vi "CCE MGLD PMJD PF SubVI02.vi"(11 "captura":T2) -> (0 "orientacion correcta":bool, 1 "y":sgl, 2 "x":sgl, 3 "etiqueta detectada":bool, 5 "Image 4":T2(plugin-control))   [LabVIEW 2020]
doc: "Ceballos Conde Emanuel Meneses Gutiérrez Luis David Pineda Méndez Job Daniel 4MV6 Sistemas de visión artificial 2022/1 \nEste vi detecta si se encuentra o no el patrón de la etiqueta ( en este caso la letra pi) en la imagen y devuelve las coordenadas en pixeles del centro de dicho patrón y determina si el patrón se encuentra en la orientación correcta gracias a su ángulo obtenido"
uses:
  <vilib>/vision/Image Controls.llb/IMAQ Image.ctl
  <vilib>/vision/NI_Vision_Development_Module.lvlib
panel:
  out "Angle":sgl
  out "Number of Matches":i32
  out "Matches (real-world)":T1(array[cluster]) {"Bounding Box"."y" format="%.2f"; "Bounding Box"."x" format="%.2f"; "Score" format="%.2f"; "Scale" format="%.2f"; "Angle" format="%.2f"; "Position"."y" format="%.2f"; "Position"."x" format="%.2f"}
  out "patron":T2(plugin-control)
  out "Image 2":T2(plugin-control)
  # "Ceballos Conde Emanuel  Meneses Gutiérrez Luis David  Pineda Méndez Job Daniel 4MV6 Sistemas de visión artificial  2022/1             SubVI02"
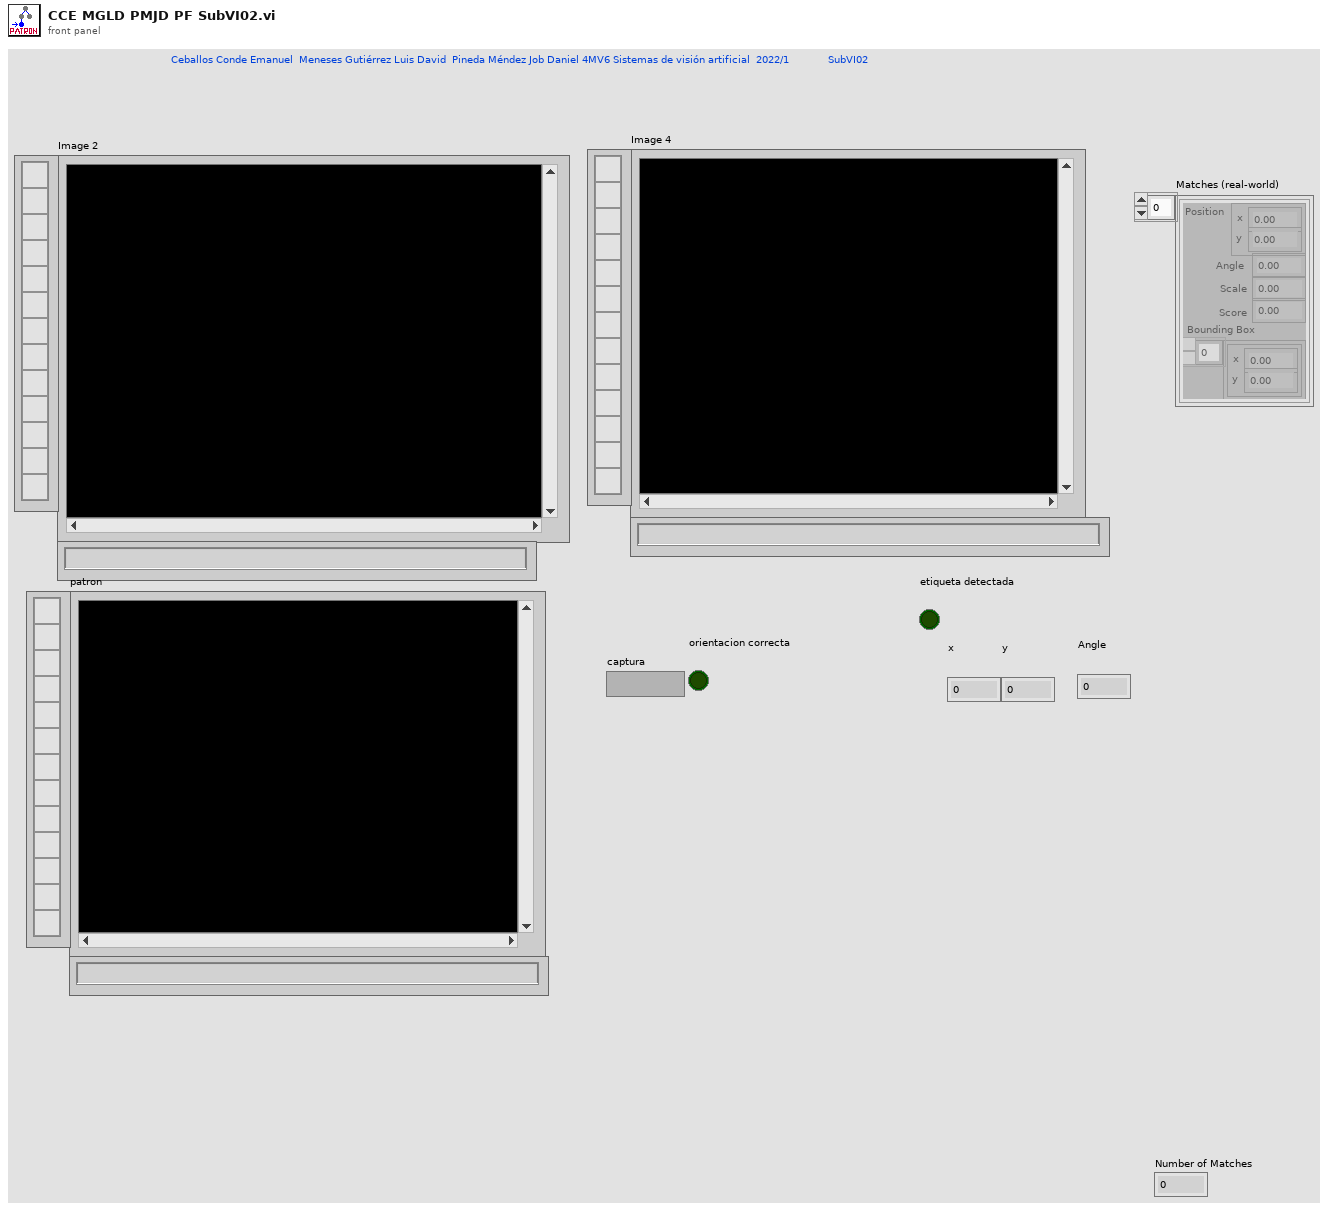
[diagram p1: front panel]
types:
  T1 = cluster{"Position":cluster{"x":sgl, "y":sgl}, "Angle":sgl, "Scale":sgl, "Score":sgl, "Bounding Box":cluster{"x":sgl, "y":sgl}[]}[]
  T2 = typedef "IMAQ Image.ctl" = refnum<image>
  T3 = cluster{"Number of Matches Requested":i32, "Minimum Match Score":sgl, "Angle Ranges":cluster{"Start Angle":sgl, "End Angle":sgl}[]}
  T4 = typedef "Image Type" = u32
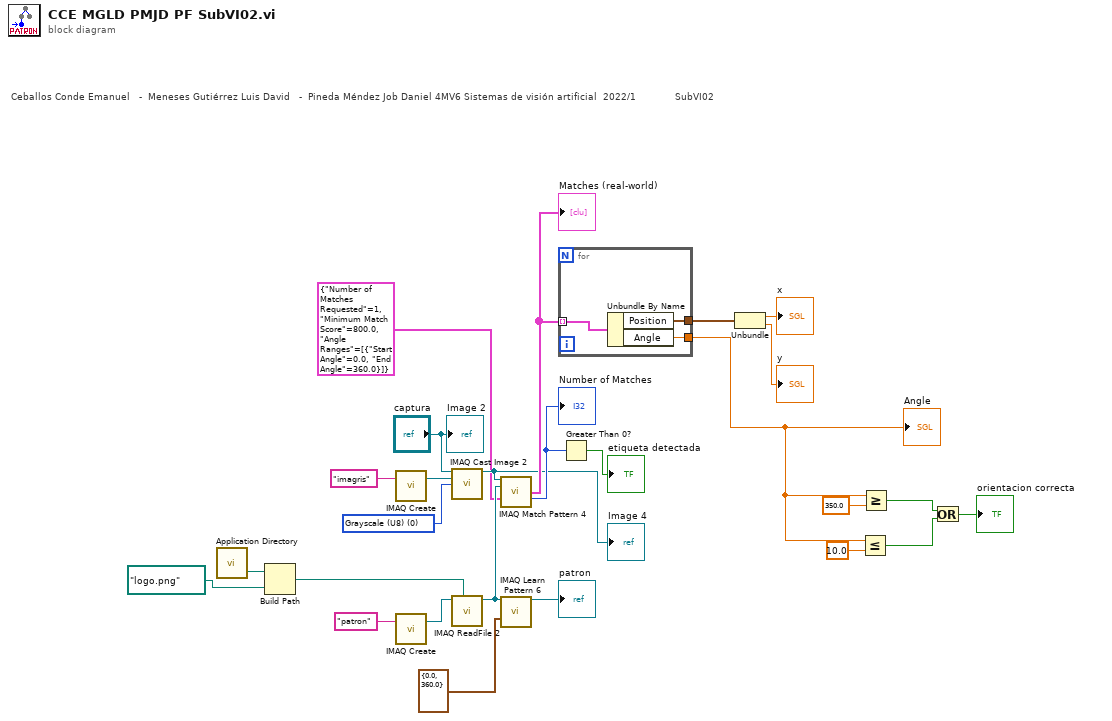
[diagram p0: block diagram]
diagram:
  w20 = T4 0 items=["Grayscale (U8)", "Grayscale (I16)", "Grayscale (SGL)", "Complex (CSG)", "RGB (U32)", "HSL (U32)", "RGB (U64)", "Grayscale (U16)"] ("Image Type")
  # "Ceballos Conde Emanuel   -  Meneses Gutiérrez Luis David   -  Pineda Méndez Job Daniel 4MV6 Sistemas de visión artificial  2022/1             SubVI02"
  n1 = call <vilib>:"Application Directory.vi"() -> ("Application Directory"=w3:path)
  n2 = Build Path(base path=w3, name or relative path=path "logo.png") -> (appended path=w1:path)
  n3 = call "IMAQ Create"("Image Name"="imagris") -> ("New Image"=w22:T2)  [unwired: 4 in, 1 out]
  n4 = call "IMAQ Create"("Image Name"="patron") -> ("New Image"=w24:T2)  [unwired: 4 in, 1 out]
  n5 = call "IMAQ Cast Image 2"("Image Src"="captura", "Image Dst"=w22, "Image Type"=w20) -> ("Image Dst Out"=w12:T2)  [unwired: 11 in, 1 out]
  "Image 4" <- w12
  n6 = call "IMAQ ReadFile 2"("File Path"=w1, "Image"=w24) -> ("Image Out"=w23:T2)  [unwired: 5 in, 4 out]
  n7 = call "IMAQ Match Pattern 4"("Image"=w12, "Template Image"=w23, "Parameters"=T3 {"Number of Matches Requested"=1, "Minimum Match Score"=800.0, "Angle Ranges"=[{"Start Angle"=0.0, "End Angle"=360.0}]}) -> ("Matches (real-world)"=w19:T1, "Number of Matches"=w18:i32)  [unwired: 8 in, 3 out]
  "Matches (real-world)" <- w19
  "Number of Matches" <- w18
  n8 = call "IMAQ Learn Pattern 6"("Image"=w23, "Angle Range"=cluster{"Start Angle":sgl, "End Angle":sgl} {"Start Angle"=0.0, "End Angle"=360.0}) -> ("Template Image Out"=→"patron":T2)  [unwired: 11 in, 2 out]
  n9 = for {
    tunnel: w19 -> [w29] mode=indexing
    tunnel: [w28] -> w16
    tunnel: [w27] -> w9
    n10 = Unbundle By Name(w29) -> ("Position"=w28:cluster{"x":sgl, "y":sgl}, "Angle"=w27:sgl)
  }
  "Angle" <- w9
  n11 = Greater Than 0?(x=w18) -> (x > 0?=→"etiqueta detectada":bool)
  n12 = Unbundle(w16) -> ("x"=→"x":sgl, "y"=→"y":sgl)
  n13 = Less Or Equal?(x=w9, y=sgl 10.0) -> (x <= y?=w7:bool)
  n14 = Greater Or Equal?(x=w9, y=sgl 350.0) -> (x >= y?=w8:bool)
  n15 = Or(x=w8, y=w7) -> (x .or. y?=→"orientacion correcta":bool)
  "Image 2" <- "captura"
